vi "Ritter Write Data.vi"(0 "Test Fixture Hardware":T23 {"Power"."Yokogawa"."WT310_3"."V Range (6: 600V)" items=["Auto", "15V", "30V", "60V", "150V", "300V", "600V"]; "Power"."Yokogawa"."WT310_3"."A Range (12: 20A)" items=["Auto", "5mA", "10mA", "20mA", "50mA", "100mA", "200mA", "0.5A", "1A", "2A", "5A", "10A", "20A", "50mV", "100mV", "200mV", "2.5V", "5V", "10V"]; "Power"."Yokogawa"."WT310_3"."Sample Rate (1: 0.25s)" items=["0.1s", "0.25s", "0.5s", "1s", "2s", "5s"]; "Power"."Yokogawa"."WT310_2"."V Range (6: 600V)" items=["Auto", "15V", "30V", "60V", "150V", "300V", "600V"]; "Power"."Yokogawa"."WT310_2"."A Range (12: 20A)" items=["Auto", "5mA", "10mA", "20mA", "50mA", "100mA", "200mA", "0.5A", "1A", "2A", "5A", "10A", "20A", "50mV", "100mV", "200mV", "2.5V", "5V", "10V"]; "Power"."Yokogawa"."WT310_2"."Sample Rate (1: 0.25s)" items=["0.1s", "0.25s", "0.5s", "1s", "2s", "5s"]; "Power"."Yokogawa"."WT500"."Update Rate (3: 500ms)" items=["-", "100ms", "200ms", "500ms", "1s", "2s", "5s"]; "Power"."Yokogawa"."WT500"."I Range (7: 40A)" items=["AUTO", "500 mA", "1 A", "2 A", "5 A", "10 A", "20 A", "40 A", "S-AUTO", "50 mV", "100 mV", "200 mV", "500 mV", "1 V", "2 V", "5 V", "10 V", "250 mA", "500 mA", "1 A", "2.5 A", "5 A", "10 A", "20 A", "25 mV", "50 mV", "100 mV", "250 mV", "500 mV", "1 V", "2.5 V", "5 V"]; "Power"."Yokogawa"."WT500"."V Range (8: 1000V)" items=["AUTO", "15", "30", "60", "100", "150", "300", "600", "1000", "7.5", "15", "30", "50", "75", "150", "300", "500"]; "Power"."Yokogawa"."WT210"."V Range (6: 600V)" items=["Auto", "15V", "30V", "60V", "150V", "300V", "600V"]; "Power"."Yokogawa"."WT210"."A Range (12: 20A)" items=["Auto", "5mA", "10mA", "20mA", "50mA", "100mA", "200mA", "0.5A", "1A", "2A", "5A", "10A", "20A", "50mV", "100mV", "200mV", "2.5V", "5V", "10V"]; "Power"."Yokogawa"."WT210"."Sample Rate (1: 0.25s)" items=["0.1s", "0.25s", "0.5s", "1s", "2s", "5s"]}, 1 "Meter Type":enum16{"Dry Meter", "Wet Meter"}(ring)=enum."Wet Meter", 5 "Core HEWH Data Input A":T1 {"Test Patten Setup"."PRAT/RLT Sequence"."Time" format="%<%H:%M:%S>t"; "Test Patten Setup"."Total Gallons Schedule" format="%.2f"}, 11 "error in (no error)":errorcluster, 12 "Ritter Gas Drum Meter":bool) -> (4 "String Data":string[][](array[string]), 6 "Core HEWH Data Output":T1 {"Test Patten Setup"."PRAT/RLT Sequence"."Time" format="%<%H:%M:%S>t"; "Test Patten Setup"."Total Gallons Schedule" format="%.2f"}, 15 "error out":errorcluster)   [LabVIEW 2023]
uses:
  Trunk/Washer DOE/Type Definitions/DOE Test Fixture Hardware.ctl
  <vilib>/NI/Modbus Library/API/Master/Modbus Master.lvclass
  Trunk/Utility/Type Definitions/UTILITY Power Inputs Control.ctl
  IND560 Scale Monitor/Type Definitions/IND560 Configuration.ctl
  Trunk/Hybrid Water Heater/Type Definitions/HEWH Agilent Cluster.ctl
  Trunk/Utility/Type Definitions/UTILITY TC Coefficients.ctl
  Omega FMA-1600A Series Gas Flow Meter/Type Definitions/FMA1600A COM Ports.ctl
  Alicat Gas Meter Driver/Sub-VIs/Data Frame.ctl
  Omega FMA-1600A Series Gas Flow Meter/Type Definitions/FMA1600A Units String.ctl
  Alicat Gas Meter Driver/Sub-VIs/Units of Measure.ctl
  Inficon Fusion Micro GC/Type Definitions/Inficon IP Address.ctl
  Trunk/Hybrid Water Heater/Type Definitions/HEWH Output Information.ctl
  Trunk/Hybrid Water Heater/Type Definitions/HEWH Draw Pattern Setup.ctl
  Trunk/Hybrid Water Heater/Type Definitions/PRAT Test.ctl
  Trunk/Utility/Save File/File Setup (Public)/Type Definition/Save File HEWH Heating Control Mode.ctl
  Trunk/Hybrid Water Heater/Support VIs/Draw Water Specific/Type Definitions/Terminate Draw Conditions.ctl
  Trunk/Hybrid Water Heater/Type Definitions/HEWH Start Conditions.ctl
  Trunk/Hybrid Water Heater/Support VIs/Draw Water Specific/Type Definitions/Check Special Condtions.ctl
  Trunk/Hybrid Water Heater/Support VIs/Draw Water Specific/Type Definitions/HEWH Special Condition Check.ctl
  Trunk/Hybrid Water Heater/Type Definitions/HEWH Draw Flag ENUM.ctl
  Trunk/Hybrid Water Heater/Type Definitions/HEWH Specific DAQ.ctl
  Trunk/Hybrid Water Heater/Type Definitions/HEWH Power Data.ctl
  Trunk/Hybrid Water Heater/Type Definitions/HEWH Power Elements.ctl
  Trunk/Utility/Type Definitions/UTILITY Power Analyzer.ctl
  Viasala Indigo 520/Type Definitions/Viasala Indigo 520 Data.ctl
  Tidal Engineering/Type Definitions/Tenney Environmental Chamber Data.ctl
  Trunk/Hybrid Water Heater/Type Definitions/HEWH Calc and Calibration.ctl
  Trunk/Utility/Save File/File Setup (Public)/Type Definition/Save File DOE LabView Program.ctl
  Trunk/Hybrid Water Heater/Custom Instrument Control/MW100/Type Definitions/Station ID Selector.ctl
  Trunk/Range/Type Definitions/RANGE ANSI Rate.ctl
  Trunk/Hybrid Water Heater/Custom Instrument Control/MW100/Type Definitions/HEWH Module 4 Relay Status.ctl
  Inficon Fusion Micro GC/Type Definitions/Inficon Data.ctl
  Alicat Gas Meter Driver/Sub-VIs/Data Cluster.ctl
  Trunk/Utility/Save File/File Setup.lvlib
panel:
  # "Totalizer Timer"
  # "Natural Gas"
  # "Propane"
  # "Draw Pattern Setup (24 Hour)"
  # "Totalizer Timer"
  # "Natural Gas"
  # "Propane"
  # "Draw Pattern Setup (24 Hour)"
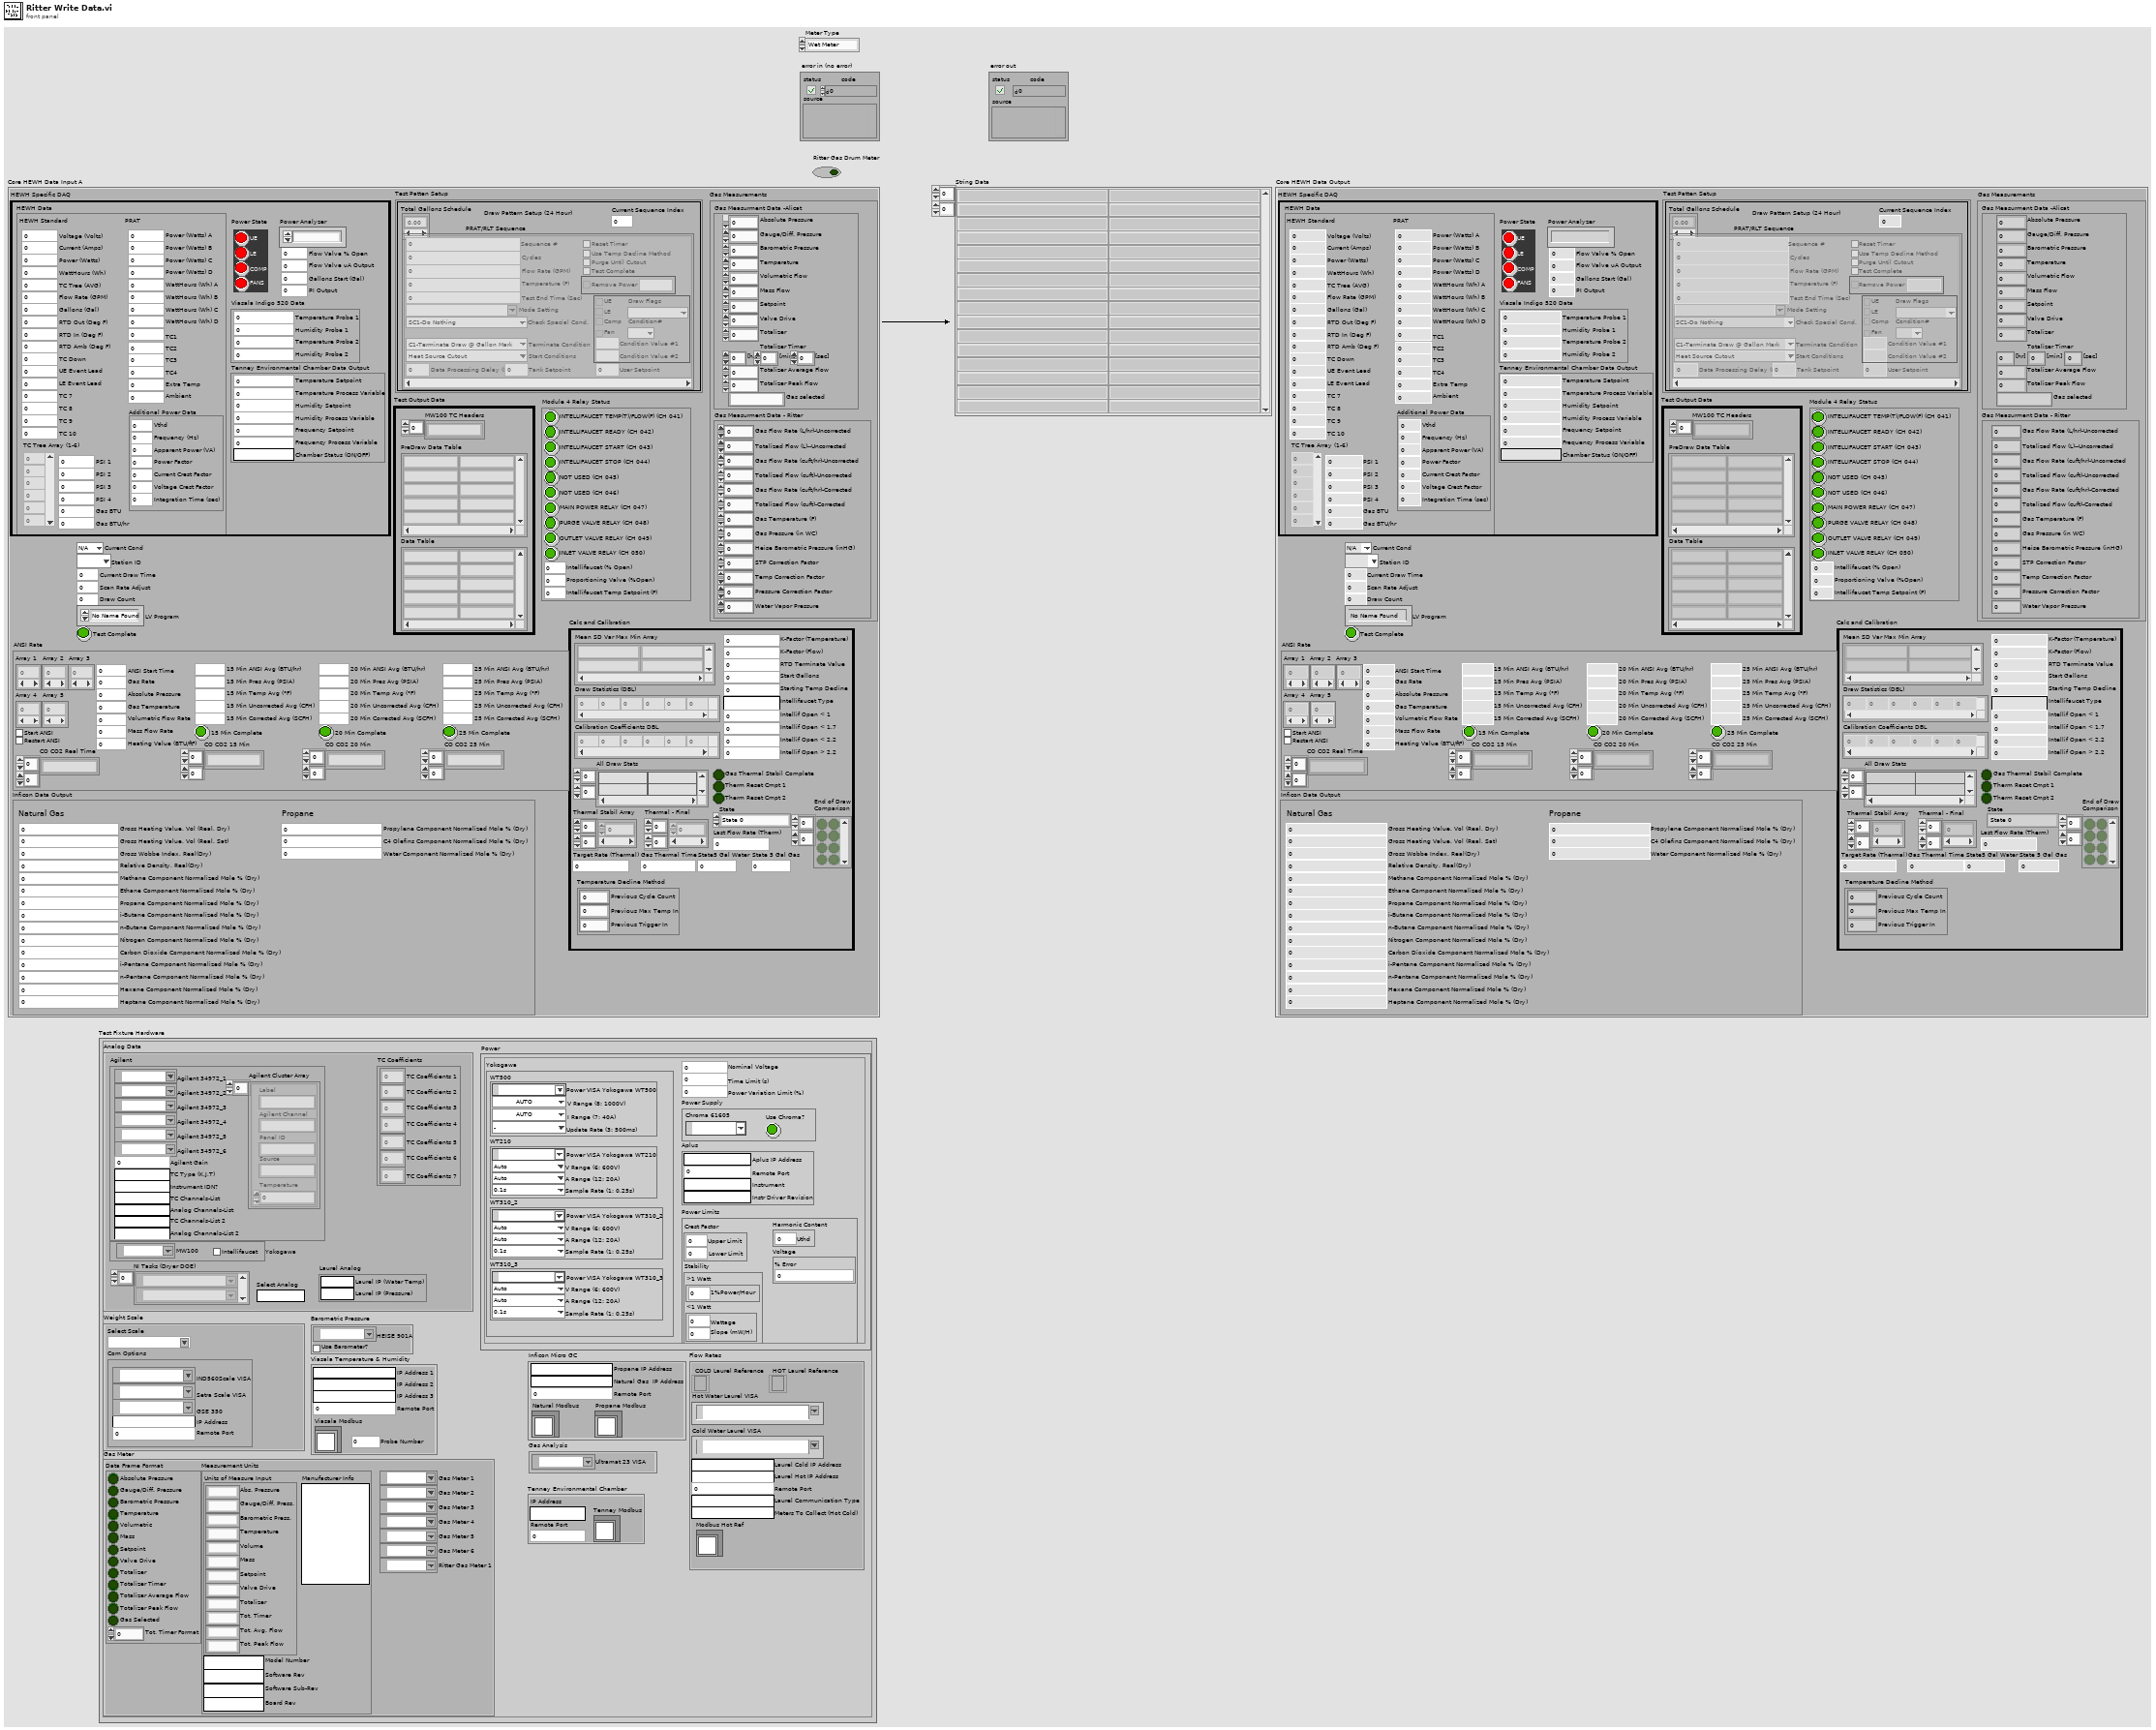
[diagram p1: front panel]
types:
  T1 = typedef "HEWH Output Information.ctl" = cluster{"Scan Rate Adjust":dbl, "Draw Count":i32, "Test Patten Setup":T2, "HEWH Specific DAQ":T10, "Test Output Data":cluster{"PreDraw Data Table":string[][], "Data Table":string[][], "MW100 TC Headers":string[]}, "Calc and Calibration":T16, "Current Draw Time":dbl, "LV Program":T17, "Station ID":T18, "Current Cond":T8, "Test Complete":bool, "ANSI Rate":T19, "Module 4 Relay Status":T20, "Inficon Data Output":T21, "Gas Measurements":cluster{"Gas Measurment Data -Alicat":T22, "Gas Measurment Data - Ritter":cluster{"Gas Flow Rate (L/hr)-Uncorrected":dbl, "Totalized Flow (L)--Uncorrected":dbl, "Gas Flow Rate (cuft/hr)-Uncorrected":dbl, "Totalized Flow (cuft)-Uncorrected":dbl, "Gas Temperature (F)":dbl, "Gas Pressure (in WC)":dbl, "Heise Barometric Pressure (inHG)":dbl, "STP Correction Factor":dbl, "Temp Correction Factor":dbl, "Pressure Correction Factor":dbl, "Water Vapor Pressure":dbl, "Gas Flow Rate (cuft/hr)-Corrected":dbl, "Totalized Flow (cuft)-Corrected":dbl}}}
  T2 = typedef "HEWH Draw Pattern Setup.ctl" = cluster{"Total Gallons Schedule":dbl[], "PRAT/RLT Sequence":T3[], "Current Sequence Index":i32}
  T3 = typedef "PRAT Test.ctl" = cluster{"Sequence #":dbl, "Cycles":i32, "Mode Setting":T4, "Flow Rate (GPM)":dbl, "Temperature (F)":dbl, "Reset Timer":bool, "Use Temp Decline Method":bool, "Terminate Condition":T5, "Condition Value #1":dbl, "UE":bool, "LE":bool, "Comp":bool, "Fan":bool, "Test End Time (Sec)":dbl, "Purge Until Cutout":bool, "Start Conditions":T6, "Condition Value #2":dbl, "Remove Power":bool, "Time":dbl, "Check Special Cond.":T7, "Condition#":T8, "Draw Flags":T9, "Data Processing Delay (FHD 15sec, UEF 5 Sec)":dbl, "Test Complete":bool, "User Setpoint":dbl, "Tank Setpoint":dbl}
  T4 = typedef "File Setup.lvlib/Save File HEWH Heating Control Mode.ctl" = string
  T5 = typedef "Terminate Draw Conditions.ctl" = enum16{"C1-Terminate Draw @ Gallon Mark", "C2-Special Last Draw (HU Test)", "C3-RTD Out <=", "C4-Mean Tank Temp <=", "C5-Decrease RTD Out (Deg F)", "C6-Time (Seconds)", "C7-Until Any Heat Source", "C8-Specific Heat Source", "C9-Do Nothing", "C10-Inlet Outlet RTD Temp Delta"}
  T6 = typedef "HEWH Start Conditions.ctl" = enum16{"Heat Source Cutout", "At Time (Seconds)", "Every X (Seconds)", "T2 >= X° Below Setpoint", "Seconds From Complete", "Wait for LE & Comp Cutout", "Wait for Comp Cutout", "Wait for LE Cutout", "Wait for UE Cutout", "Start Immediately"}
  T7 = typedef "Check Special Condtions.ctl" = enum16{"SC1-Do Nothing", "SC2-Check Heat Source (On-C2/Off-C1)", "SC3-Check Skip Condition", "SC4-Check Heat Source ON/Fail", "SC5-Keep Draw Valves Open", "SC6-Skip Purge"}
  T8 = typedef "HEWH Special Condition Check.ctl" = enum16{"N/A", "C1", "C2", "Reset/Fail", "Skip Draw Sequence"}
  T9 = typedef "HEWH Draw Flag ENUM.ctl" = enum16{"N/A", "None(0)", "Sml(1)", "Med(2)", "SmlMed(3)", "Lrg(4)", "SmlLrg(5)", "MedLrg(6)", "SmlMedLrg(7)"}
  T10 = typedef "HEWH Specific DAQ.ctl" = cluster{"HEWH Data":T11, "Flow Valve % Open":dbl, "Power State":T12, "Power Analyzer":T13, "Flow Valve uA Output":i32, "Gallons Start (Gal)":dbl, "PI Output":dbl, "Viasala Indigo 520 Data":T14, "Tenney Environmental Chamber Data Output":T15}
  T11 = typedef "HEWH Power Data.ctl" = cluster{"HEWH Standard":cluster{"Voltage (Volts)":dbl, "Current (Amps)":dbl, "Power (Watts)":dbl, "WattHours (Wh)":dbl, "TC Tree (AVG)":dbl, "Flow Rate (GPM)":dbl, "Gallons (Gal)":dbl, "RTD Out (Deg F)":dbl, "RTD In (Deg F)":dbl, "RTD Amb (Deg F)":dbl, "TC Down":dbl, "UE Event Lead":i32, "LE Event Lead":i32, "TC 8":dbl, "TC 9":dbl, "TC 10":dbl, "TC Tree Array (1-6)":dbl[], "TC 7":dbl, "PSI 1":dbl, "PSI 2":dbl, "PSI 3":dbl, "PSI 4":dbl, "Gas BTU":dbl, "Gas BTU/hr":dbl}, "PRAT":cluster{"Power (Watts) A":dbl, "Power (Watts) B":dbl, "Power (Watts) C":dbl, "Power (Watts) D":dbl, "TC1":dbl, "TC2":dbl, "TC3":dbl, "TC4":dbl, "WattHours (Wh) A":dbl, "WattHours (Wh) B":dbl, "WattHours (Wh) C":dbl, "WattHours (Wh) D":dbl, "Ambient":dbl, "Extra Temp":dbl}, "Additional Power Data":cluster{"Vthd":dbl, "Frequency (Hz)":dbl, "Apparent Power (VA)":dbl, "Power Factor":dbl, "Current Crest Factor":dbl, "Voltage Crest Factor":dbl, "Integration Time (sec)":dbl}}
  T12 = typedef "HEWH Power Elements.ctl" = cluster{"UE":bool, "LE":bool, "COMP":bool, "FANS":bool}
  T13 = typedef "UTILITY Power Analyzer.ctl" = enum16{"", "APLUS", "WT210", "WT500", "WT300", "OSI", "Debug", "WT230", "WT300_1", "WT300_2"}
  T14 = typedef "Viasala Indigo 520 Data.ctl" = cluster{"Temperature Probe 1":dbl, "Humidity Probe 1":dbl, "Temperature Probe 2":dbl, "Humidity Probe 2":dbl}
  T15 = typedef "Tenney Environmental Chamber Data.ctl" = cluster{"Temperature Setpoint":dbl, "Temperature Process Variable":dbl, "Humidity Setpoint":dbl, "Humidity Process Variable":dbl, "Frequency Setpoint":dbl, "Frequency Process Variable":dbl, "Chamber Status (ON/OFF)":string}
  T16 = typedef "HEWH Calc and Calibration.ctl" = cluster{"Mean SD Var Max Min Array":string[][], "Draw Statistics (DBL)":dbl[][], "Calibration Coefficients DBL":dbl[][], "Start Gallons":dbl, "Starting Temp Decline":dbl, "K-Factor (Temperature)":dbl, "All Draw Stats":string[][], "RTD Terminate Value":dbl, "K-Factor (Flow)":dbl, "Intellifaucet Type":string, "Thermal Stabil Array":dbl[][], "Gas Thermal Stabil Complete":bool, "Therm Reset Cmpt 1":bool, "Therm Reset Cmpt 2":bool, "Last Flow Rate (Therm)":dbl, "State":enum16{"State 0", "State 1", "State 2", "State 3", "State 4", "State 5", "State 6"}, "Gas Thermal Time":dbl, "Target Rate (Thermal)":dbl, "Thermal - Final":dbl[][], "State5 Gal Water":dbl, "State 5 Gal Gas":dbl, "Intellif Open < 1":dbl, "Intellif Open < 1.7":dbl, "Intellif Open < 2.2":dbl, "Intellif Open > 2.2":dbl, "End of Draw\nComparison":bool[][], "Temperature Decline Method":cluster{"Previous Cycle Count":i32, "Previous Max Temp In":dbl, "Previous Trigger In":u8}}
  T17 = typedef "File Setup.lvlib/Save File DOE LabView Program.ctl" = enum16{"No Name Found", "DOE Stand", "Dishwasher Kitchen", "Portable Stand", "HEWH", "Dryer", "Dryer WILT", "HCC", "PRAT", "HEWH RLT", "Refrigeration", "Gas Water Heater"}
  T18 = typedef "Station ID Selector.ctl" = enum16{"", "A", "B", "C", "D", "Global"}
  T19 = typedef "RANGE ANSI Rate.ctl" = cluster{"Array 1":dbl[], "Array 3":dbl[], "Array 2":dbl[], "Start ANSI":bool, "ANSI Start Time":dbl, "Restart ANSI":bool, "15 Min ANSI Avg (BTU/hr)":dbl, "20 Min ANSI Avg (BTU/hr)":dbl, "25 Min ANSI Avg (BTU/hr)":dbl, "Absolute Pressure":dbl, "Gas Temperature":dbl, "Volumetric Flow Rate":dbl, "Mass Flow Rate":dbl, "Array 4":dbl[], "Array 5":dbl[], "Gas Rate":dbl, "15 Min Pres Avg (PSIA)":dbl, "20 Min Pres Avg (PSIA)":dbl, "25 Min Pres Avg (PSIA)":dbl, "15 Min Temp Avg (°F) ":dbl, "20 Min Temp Avg (°F)":dbl, "25 Min Temp Avg (°F)":dbl, "15 Min Uncorrected Avg (CFH)":dbl, "20 Min Uncorrected Avg (CFH)":dbl, "25 Min Uncorrected Avg (CFH)":dbl, "15 Min Corrected Avg (SCFH)":dbl, "20 Min Corrected Avg (SCFH)":dbl, "25 Min Corrected Avg (SCFH)":dbl, "15 Min Complete":bool, "20 Min Complete":bool, "25 Min Complete":bool, "Heating Value (BTU/ft³)":dbl, "CO CO2 15 Min":string[][], "CO CO2 20 Min":string[][], "CO CO2 25 Min":string[][], "CO CO2 Real Time":string[][]}
  T20 = typedef "HEWH Module 4 Relay Status.ctl" = cluster{"INTELLIFAUCET TEMP(T)/FLOW(F) (CH 041)":bool, "INTELLIFAUCET READY (CH 042)":bool, "INTELLIFAUCET START (CH 043)":bool, "INTELLIFAUCET STOP (CH 044)":bool, "MAIN POWER RELAY (CH 047)":bool, "NOT USED (CH 045)":bool, "NOT USED (CH 046)":bool, "PURGE VALVE RELAY (CH 048)":bool, "OUTLET VALVE RELAY (CH 049)":bool, "INLET VALVE RELAY (CH 050)":bool, "Intellifaucet (% Open)":dbl, "Proportioning Valve (%Open)":dbl, "Intellifaucet Temp Setpoint (F)":dbl}
  T21 = typedef "Inficon Data.ctl" = cluster{"Gross Heating Value, Vol (Real, Dry)":dbl, "Nitrogen Component Normalized Mole % (Dry)":dbl, "Methane Component Normalized Mole % (Dry)":dbl, "Carbon Dioxide Component Normalized Mole % (Dry)":dbl, "Ethane Component Normalized Mole % (Dry)":dbl, "Propane Component Normalized Mole % (Dry)":dbl, "i-Pentane Component Normalized Mole % (Dry)":dbl, "i-Butane Component Normalized Mole % (Dry)":dbl, "n-Butane Component Normalized Mole % (Dry)":dbl, "n-Pentane Component Normalized Mole % (Dry)":dbl, "Hexane Component Normalized Mole % (Dry)":dbl, "Heptane Component Normalized Mole % (Dry)":dbl, "Gross Wobbe Index, Real(Dry)":dbl, "Relative Density, Real(Dry)":dbl, "Propylene Component Normalized Mole % (Dry)":dbl, "C4 Olefins Component Normalized Mole % (Dry)":dbl, "Water Component Normalized Mole % (Dry)":dbl, "Gross Heating Value, Vol (Real, Sat)":dbl}
  T22 = typedef "Data Cluster.ctl" = cluster{"Absolute Pressure":dbl, "Gauge/Diff. Pressure":dbl, "Barometric Pressure":dbl, "Temperature":dbl, "Volumetric Flow":dbl, "Mass Flow":dbl, "Setpoint":dbl, "Valve Drive":dbl, "Totalizer":dbl, "[hr]":dbl, "[min]":dbl, "[sec]":dbl, "Totalizer Average Flow":dbl, "Totalizer Peak Flow":dbl, "Gas selected":string}
  T23 = typedef "DOE Test Fixture Hardware.ctl" = cluster{"Power ":T24, "Weight Scale":cluster{"Com Options":T25, "Select Scale":string}, "Flow Rates":cluster{"Laurel Cold IP Address":string, "Laurel Hot IP Address":string, "Hot Water Laurel VISA":refnum<visa-resource-name>, "Cold Water Laurel VISA":refnum<visa-resource-name>, "Remote Port":u16, "Laurel Communication Type":string, "Meters To Collect (Hot Cold)":string, "HOT Laurel Reference":refnum<k5>, "COLD Laurel Reference":refnum<k5>, "Modbus Hot Ref":refnum<class "Modbus Master.lvclass">}, "Analog Data":cluster{"Agilent":cluster{"Agilent 34972_1":refnum<visa-resource-name>, "Agilent 34972_2":refnum<visa-resource-name>, "Agilent 34972_3":refnum<visa-resource-name>, "Agilent 34972_4":refnum<visa-resource-name>, "Agilent 34972_5":refnum<visa-resource-name>, "Agilent 34972_6":refnum<visa-resource-name>, "Agilent Gain":dbl, "TC Type (K,J,T)":string, "Instrument IDN?":string, "TC Channels-List":string, "Analog Channels-List":string, "Agilent Cluster Array":T26[], "TC Channels-List 2":string, "Analog Channels-List 2":string}, "Yokogawa":cluster{"MW100":refnum<visa-resource-name>, "Intellifaucet":bool}, "Select Analog":string, "TC Coefficients":T27, "NI Tasks (Dryer DOE)":refnum<k21>[], "Laurel Analog":cluster{"Laurel IP (Water Temp)":string, "Laurel IP (Pressure)":string}}, "Viasala Temperature & Humidity":cluster{"IP Address 1":string, "Remote Port":u16, "IP Address 2":string, "IP Address 3":string, "Viasala Modbus":refnum<class "Modbus Master.lvclass">, "Probe Number":u16}, "Gas Meter":T28, "Barometric Pressure":cluster{"HEISE 901A":refnum<visa-resource-name>, "Use Barometer?":bool}, "Gas Analysis":cluster{"Ultramat 23 VISA":refnum<visa-resource-name>}, "Inficon Micro GC":T32, "Tenney Environmental Chamber":cluster{"Remote Port":u16, "IP Address":string, "Tenney Modbus":refnum<class "Modbus Master.lvclass">}}
  T24 = typedef "UTILITY Power Inputs Control.ctl" = cluster{"Yokogawa":cluster{"WT210":cluster{"Sample Rate (1: 0.25s)":i32, "A Range (12: 20A)":i32, "V Range (6: 600V)":i32, "Power VISA Yokogawa WT210":refnum<visa-resource-name>}, "WT500":cluster{"Power VISA Yokogawa WT500":refnum<visa-resource-name>, "V Range (8: 1000V)":i32, "I Range (7: 40A)":i32, "Update Rate (3: 500ms)":i32}, "WT310_2":cluster{"Sample Rate (1: 0.25s)":i32, "A Range (12: 20A)":i32, "V Range (6: 600V)":i32, "Power VISA Yokogawa WT310_2":refnum<visa-resource-name>}, "WT310_3":cluster{"Sample Rate (1: 0.25s)":i32, "A Range (12: 20A)":i32, "V Range (6: 600V)":i32, "Power VISA Yokogawa WT310_3":refnum<visa-resource-name>}}, "Aplus":cluster{"Aplus IP Address":string, "Remote Port":i32, "Instrument":string, "Instr Driver Revision":string}, "Power Limits":cluster{"Crest Factor":cluster{"Upper Limit":dbl, "Lower Limit":dbl}, "Harmonic Content":cluster{"Uthd":dbl}, "Voltage":cluster{"% Error":dbl}, "Stability":cluster{"<1 Watt ":cluster{"Wattage":dbl, "Slope (mW/H)":dbl}, ">1 Watt":cluster{"1%Power/Hour":dbl}}}, "Nominal Voltage":i32, "Time Limit (s)":dbl, "Power Variation Limit (%)":dbl, "Power Supply":cluster{"Chroma 61605":refnum<visa-resource-name>, "Use Chroma?":bool}}
  T25 = typedef "IND560 Configuration.ctl" = cluster{"IND560Scale VISA":refnum<visa-resource-name>, "IP Address":string, "Remote Port":u16, "Setra Scale VISA":refnum<visa-resource-name>, "GSE 350":refnum<visa-resource-name>}
  T26 = typedef "HEWH Agilent Cluster.ctl" = cluster{"Label":string, "Agilent Channel":string, "Panel ID":string, "Source":string, "Temperature":dbl}
  T27 = typedef "UTILITY TC Coefficients.ctl" = cluster{"TC Coefficients 1":dbl[], "TC Coefficients 2":dbl[], "TC Coefficients 3":dbl[], "TC Coefficients 4":dbl[], "TC Coefficients 5":dbl[], "TC Coefficients 6":dbl[], "TC Coefficients 7":dbl[]}
  T28 = typedef "FMA1600A COM Ports.ctl" = cluster{"Gas Meter 1":refnum<visa-resource-name>, "Gas Meter 2":refnum<visa-resource-name>, "Gas Meter 3":refnum<visa-resource-name>, "Gas Meter 4":refnum<visa-resource-name>, "Gas Meter 5":refnum<visa-resource-name>, "Gas Meter 6":refnum<visa-resource-name>, "Data Frame Format":T29, "Measurement Units":T30, "Ritter Gas Meter 1":refnum<visa-resource-name>}
  T29 = typedef "Data Frame.ctl" = cluster{"Absolute Pressure":bool, "Gauge/Diff. Pressure":bool, "Barometric Pressure":bool, "Temperature":bool, "Volumetric":bool, "Mass":bool, "Setpoint":bool, "Valve Drive":bool, "Totalizer":bool, "Totalizer Timer":bool, "Totalizer Average Flow":bool, "Totalizer Peak Flow":bool, "Gas Selected":bool, "Tot. Timer Format":u16}
  T30 = typedef "FMA1600A Units String.ctl" = cluster{"Software Rev":string, "Model Number":string, "Manufacturer Info":string, "Software Sub-Rev":string, "Board Rev":string, "Units of Measure Input":T31}
  T31 = typedef "Units of Measure.ctl" = cluster{"Abs. Pressure":string, "Gauge/Diff. Press.":string, "Barometric Press.":string, "Temperature":string, "Volume":string, "Mass":string, "Setpoint":string, "Valve Drive":string, "Totalizer":string, "Tot. Timer":string, "Tot. Avg. Flow":string, "Tot. Peak Flow":string}
  T32 = typedef "Inficon IP Address.ctl" = cluster{"Propane IP Address":string, "Natural Gas  IP Address":string, "Remote Port":u16, "Natural Modbus":refnum<class "Modbus Master.lvclass">, "Propane Modbus":refnum<class "Modbus Master.lvclass">}
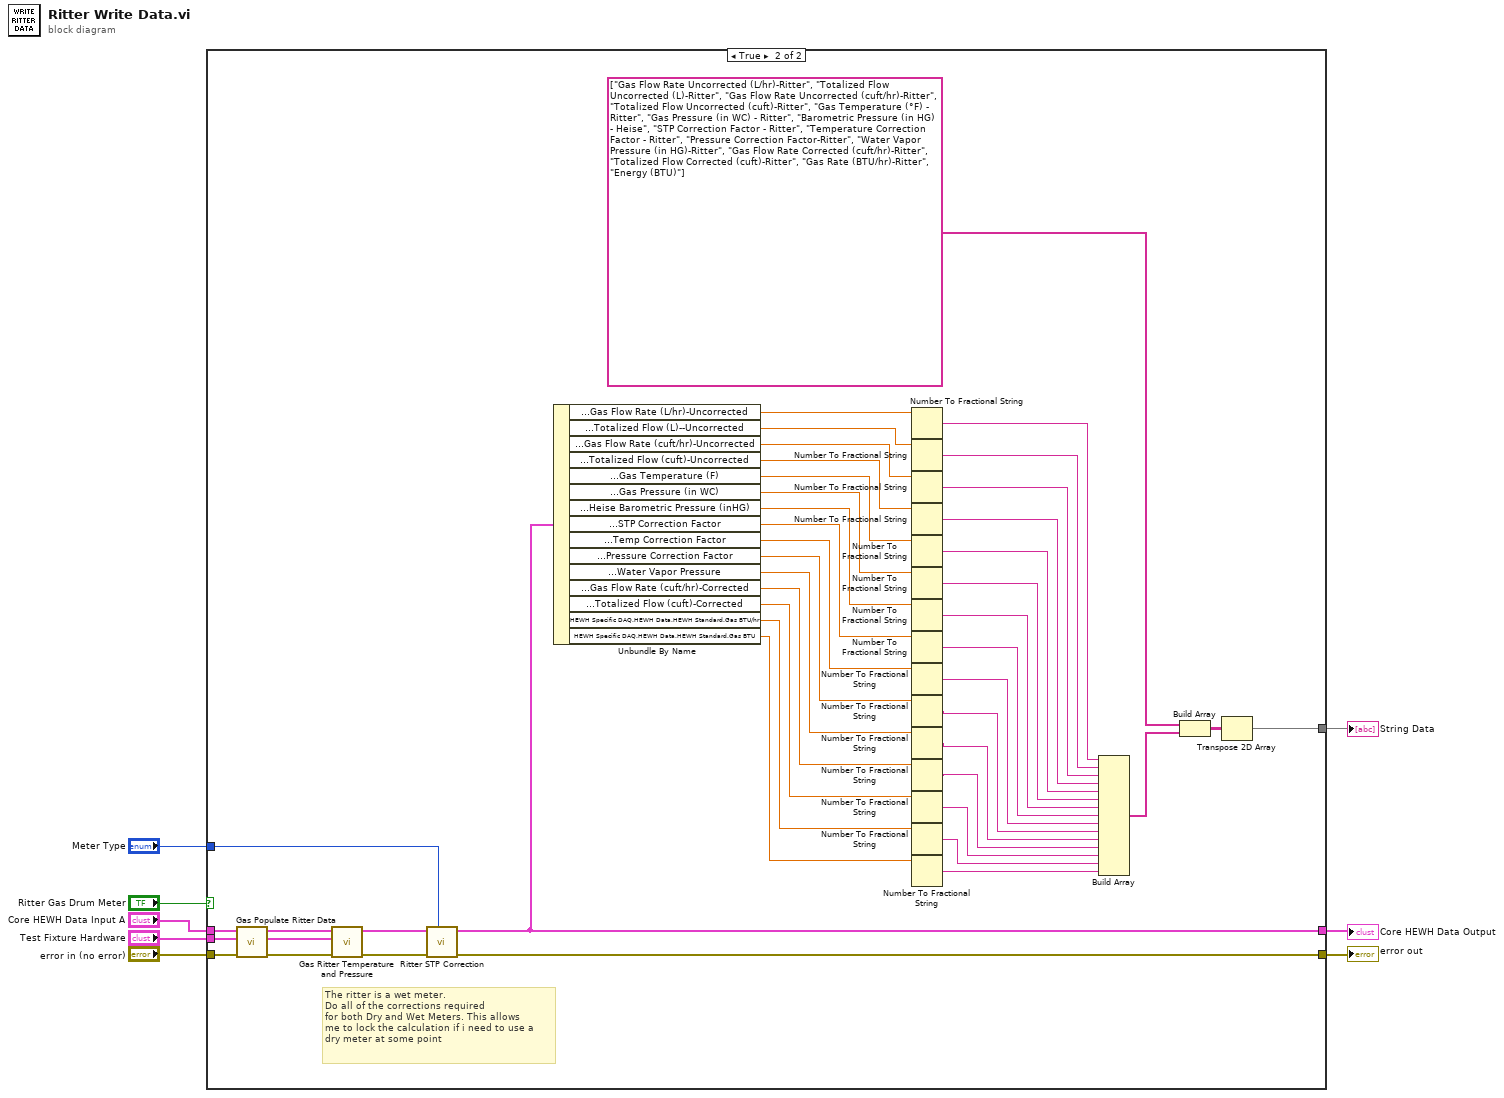
[diagram p0: block diagram]
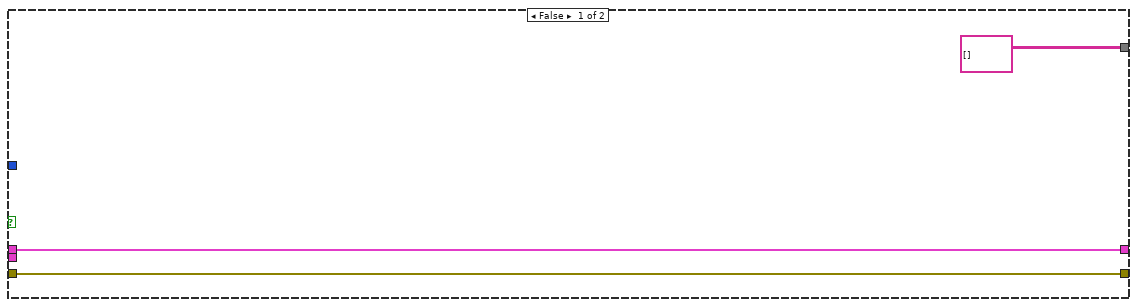
[diagram p2: hidden frame]
diagram:
  n1 = case shown="True" "Ritter Gas Drum Meter" {
    tunnel: "error in (no error)" -> [w11 w54]
    tunnel: "Test Fixture Hardware" -> [_ w53]
    tunnel: [w11 w41] -> w6
    tunnel: "Core HEWH Data Input A" -> [w9 w40]
    tunnel: [w9 w38] -> w2
    tunnel: [string[][] [] w37] -> w3
    tunnel: "Meter Type" -> [_ w12]
    frame False {
    }
    frame True {
      # "The ritter is a wet meter. \nDo all of the corrections required\nfor both Dry and Wet Meters. This allows\nme to lock the calculation if i need to use a \ndry meter at some point"
      n2 = call "Gas Populate Ritter Data.vi"("error in (no error)"=w54, "Test Fixture Hardware"=w53, "Core HEWH Data Input A"=w40) -> ("error out"=w45:errorcluster, "Test Fixture Hardware Output"=w13:T23, "Core HEWH Data Output"=w44:T1)  [unwired: 6 in]
      n3 = call "Gas Ritter Temperature and Pressure.vi"("error in (no error)"=w45, "Test Fixture Hardware"=w13, "Core HEWH Data Input A"=w44) -> ("error out"=w43:errorcluster, "Core HEWH Data Output"=w42:T1)  [unwired: 7 in]
      n4 = call "Ritter STP Correction.vi"("Meter Type"=w12, "error in"=w43, "Core HEWH Data Input A"=w42) -> ("error out"=w41:errorcluster, "Core HEWH Data Output"=w38:T1)  [unwired: 7 in]
      n5 = Unbundle By Name(w38) -> ("Gas Measurements.Gas Measurment Data - Ritter.Gas Flow Rate (L/hr)-Uncorrected"=w35:dbl, "Gas Measurements.Gas Measurment Data - Ritter.Totalized Flow (L)--Uncorrected"=w34:dbl, "Gas Measurements.Gas Measurment Data - Ritter.Gas Flow Rate (cuft/hr)-Uncorrected"=w33:dbl, "Gas Measurements.Gas Measurment Data - Ritter.Totalized Flow (cuft)-Uncorrected"=w32:dbl, "Gas Measurements.Gas Measurment Data - Ritter.Gas Temperature (F)"=w31:dbl, "Gas Measurements.Gas Measurment Data - Ritter.Gas Pressure (in WC)"=w30:dbl, "Gas Measurements.Gas Measurment Data - Ritter.Heise Barometric Pressure (inHG)"=w29:dbl, "Gas Measurements.Gas Measurment Data - Ritter.STP Correction Factor"=w28:dbl, "Gas Measurements.Gas Measurment Data - Ritter.Temp Correction Factor"=w27:dbl, "Gas Measurements.Gas Measurment Data - Ritter.Pressure Correction Factor"=w26:dbl, "Gas Measurements.Gas Measurment Data - Ritter.Water Vapor Pressure"=w25:dbl, "Gas Measurements.Gas Measurment Data - Ritter.Gas Flow Rate (cuft/hr)-Corrected"=w24:dbl, "Gas Measurements.Gas Measurment Data - Ritter.Totalized Flow (cuft)-Corrected"=w23:dbl, "HEWH Specific DAQ.HEWH Data.HEWH Standard.Gas BTU/hr"=w22:dbl, "HEWH Specific DAQ.HEWH Data.HEWH Standard.Gas BTU"=w21:dbl)
      n6 = Number To Fractional String(number=w35) -> (F-format string=w52:string)  [unwired: 3 in]
      n7 = Number To Fractional String(number=w34) -> (F-format string=w51:string)  [unwired: 3 in]
      n8 = Number To Fractional String(number=w33) -> (F-format string=w50:string)  [unwired: 3 in]
      n9 = Number To Fractional String(number=w32) -> (F-format string=w49:string)  [unwired: 3 in]
      n10 = Number To Fractional String(number=w31) -> (F-format string=w48:string)  [unwired: 3 in]
      n11 = Number To Fractional String(number=w30) -> (F-format string=w47:string)  [unwired: 3 in]
      n12 = Number To Fractional String(number=w29) -> (F-format string=w39:string)  [unwired: 3 in]
      n13 = Number To Fractional String(number=w28) -> (F-format string=w46:string)  [unwired: 3 in]
      n14 = Number To Fractional String(number=w27) -> (F-format string=w20:string)  [unwired: 3 in]
      n15 = Number To Fractional String(number=w26) -> (F-format string=w19:string)  [unwired: 3 in]
      n16 = Number To Fractional String(number=w25) -> (F-format string=w18:string)  [unwired: 3 in]
      n17 = Number To Fractional String(number=w24) -> (F-format string=w17:string)  [unwired: 3 in]
      n18 = Number To Fractional String(number=w23) -> (F-format string=w16:string)  [unwired: 3 in]
      n19 = Number To Fractional String(number=w22) -> (F-format string=w15:string)  [unwired: 3 in]
      n20 = Number To Fractional String(number=w21) -> (F-format string=w14:string)  [unwired: 3 in]
      n21 = Build Array(w52, w51, w50, w49, w48, w47, w39, w46, w20, w19, w18, w17, w16, w15, w14) -> (w56:string[])
      n22 = Build Array(string[] ["Gas Flow Rate Uncorrected (L/hr)-Ritter", "Totalized Flow Uncorrected (L)-Ritter", "Gas Flow Rate Uncorrected (cuft/hr)-Ritter", "Totalized Flow Uncorrected (cuft)-Ritter", "Gas Temperature (°F) - Ritter", "Gas Pressure (in WC) - Ritter", "Barometric Pressure (in HG) - Heise", "STP Correction Factor - Ritter", "Temperature Correction Factor - Ritter", "Pressure Correction Factor-Ritter", "Water Vapor Pressure (in HG)-Ritter", "Gas Flow Rate Corrected (cuft/hr)-Ritter", "Totalized Flow Corrected (cuft)-Ritter", "Gas Rate (BTU/hr)-Ritter", "Energy (BTU)"] ("appended array 2"), w56) -> (w55:string[][])
      n23 = Transpose 2D Array(2D array=w55) -> (transposed array=w37:string[][])
    }
  }
  "error out" <- w6
  "String Data" <- w3
  "Core HEWH Data Output" <- w2
